vi "datacomb.vi"(0 "object in":refnum<class "212format_work.lvclass">, 1 "枚举":T1(ring), 5 "error in (no error)":errorcluster) -> (14 "object out":refnum<class "212format_work.lvclass">, 15 "字符串":string, 19 "error out":errorcluster)   [LabVIEW 2016, in "212format_work.lvclass"]
uses:
  212format_work.lvclass
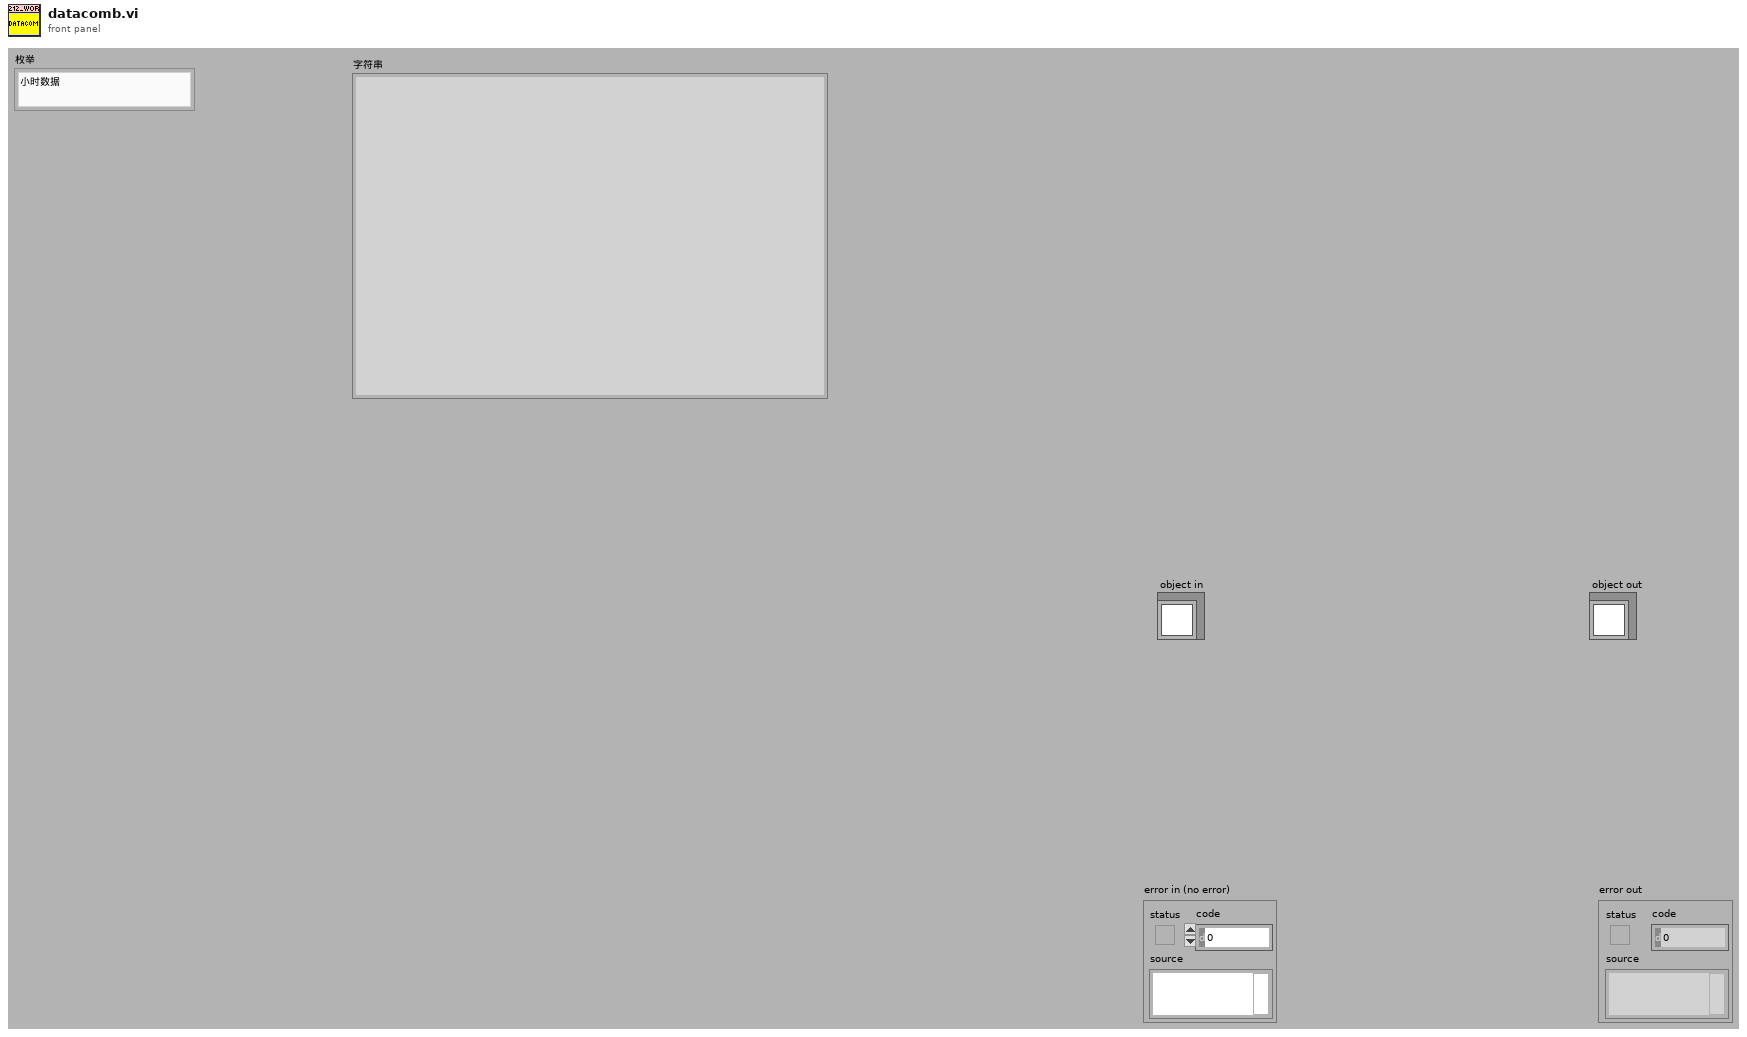
[diagram p1: front panel]
types:
  T1 = enum16{"小时数据", "实时数据", "平行样测试", "集成干预测试", "加标回收测试", "核查数据", "空白零点跨度数据", "提取小时数据", "提取实时数据", "操作日志", "仪器参数", "3090仪器参数", "提取仪器参数", "报警信息"}
  T2 = typedef "212format_work.lvclass/data控件.ctl" = cluster{"选择发送的参数":string, "插值后的数组元素":cluster{"PH":string[][], "CODCr":string[][], "氨氮":string[][], "CODMn":string[][], "总氮":string[][], "总磷":string[][], "电导率":string[][], "水温":string[][], "DO":string[][], "浊度":string[][], "叶绿素":string[][], "藻密度":string[][], "铜":string[][], "盐度":string[][], "水位":string[][], "流速":string[][], "瞬时流量":string[][], "累积流量":string[][], "亚硝酸盐":string[][], "硫化物":string[][], "ORP":string[][], "铅":string[][], "镉":string[][], "锌":string[][], "镍":string[][], "锰":string[][], "汞":string[][], "气温":string[][], "气压":string[][], "风速":string[][], "风向":string[][], "盐度 2":string[][], "磷酸盐":string[][], "硝氮":string[][], "氟化物":string[][], "挥发酚":string[][], "氯化物":string[][]}, "register values":u16[], "columns输出":string[], "环境参数":string[][], "仪器编码":string, "实时数据发送间隔":u32, "实时数据参数":string, "参数系数簇":cluster{"CODMn":dbl, "CODCr":dbl, "DO":dbl, "铜":dbl, "PH":dbl, "氨氮":dbl, "比电导率":dbl, "水温":dbl, "COD":dbl, "浊度":dbl, "总氮":dbl, "总磷":dbl, "叶绿素a":dbl, "藻密度":dbl, "水位":dbl, "流速":dbl, "瞬时流量":dbl, "累积流量":dbl, "亚硝酸盐":dbl, "硫化物":dbl, "ORP":dbl, "铅":dbl, "镉":dbl, "锌":dbl, "镍":dbl, "锰":dbl, "汞":dbl, "气温":dbl, "气压":dbl, "风速":dbl, "风向":dbl, "盐度":dbl, "磷酸盐":dbl, "硝氮":dbl, "氟化物":dbl, "挥发酚":dbl, "氯化物":dbl}, "因子编码簇":cluster{"CODMn":string, "CODCr":string, "DO":string, "铜":string, "PH":string, "氨氮":string, "比电导率":string, "水温":string, "COD":string, "浊度":string, "总氮":string, "总磷":string, "叶绿素a":string, "藻密度":string, "水位":string, "流速":string, "瞬时流量":string, "累积流量":string, "亚硝酸盐":string, "硫化物":string, "ORP":string, "铅":string, "镉":string, "锌":string, "镍":string, "锰":string, "汞":string, "气温":string, "气压":string, "风速":string, "风向":string, "盐度":string, "磷酸盐":string, "硝氮":string, "氟化物":string, "挥发酚":string, "氯化物":string}, "小时数据发送次数":i32, "读取试剂余量的值":u16[], "参数编码":string, "数据数组大小":i32, "总包数":i32, "当前包号":i32, "columns":string[], "剖面多参数":string[][], "分包标准":i32}
  T3 = cluster{"PH":string[][], "CODCr":string[][], "氨氮":string[][], "CODMn":string[][], "总氮":string[][], "总磷":string[][], "电导率":string[][], "水温":string[][], "DO":string[][], "浊度":string[][], "叶绿素":string[][], "藻密度":string[][], "铜":string[][], "盐度":string[][], "水位":string[][], "流速":string[][], "瞬时流量":string[][], "累积流量":string[][], "亚硝酸盐":string[][], "硫化物":string[][], "ORP":string[][], "铅":string[][], "镉":string[][], "锌":string[][], "镍":string[][], "锰":string[][], "汞":string[][], "气温":string[][], "气压":string[][], "风速":string[][], "风向":string[][], "盐度 2":string[][], "磷酸盐":string[][], "硝氮":string[][], "氟化物":string[][], "挥发酚":string[][], "氯化物":string[][]}
  T4 = cluster{"CODMn":dbl, "CODCr":dbl, "DO":dbl, "铜":dbl, "PH":dbl, "氨氮":dbl, "比电导率":dbl, "水温":dbl, "COD":dbl, "浊度":dbl, "总氮":dbl, "总磷":dbl, "叶绿素a":dbl, "藻密度":dbl, "水位":dbl, "流速":dbl, "瞬时流量":dbl, "累积流量":dbl, "亚硝酸盐":dbl, "硫化物":dbl, "ORP":dbl, "铅":dbl, "镉":dbl, "锌":dbl, "镍":dbl, "锰":dbl, "汞":dbl, "气温":dbl, "气压":dbl, "风速":dbl, "风向":dbl, "盐度":dbl, "磷酸盐":dbl, "硝氮":dbl, "氟化物":dbl, "挥发酚":dbl, "氯化物":dbl}
  T5 = cluster{"CODMn":string, "CODCr":string, "DO":string, "铜":string, "PH":string, "氨氮":string, "比电导率":string, "水温":string, "COD":string, "浊度":string, "总氮":string, "总磷":string, "叶绿素a":string, "藻密度":string, "水位":string, "流速":string, "瞬时流量":string, "累积流量":string, "亚硝酸盐":string, "硫化物":string, "ORP":string, "铅":string, "镉":string, "锌":string, "镍":string, "锰":string, "汞":string, "气温":string, "气压":string, "风速":string, "风向":string, "盐度":string, "磷酸盐":string, "硝氮":string, "氟化物":string, "挥发酚":string, "氯化物":string}
  T6 = typedef "212format_work.lvclass/interdata控件.ctl" = cluster{"数据发送协议":enum16{"2005-212协议", "2017-212协议"}, "枚举":enum16{"返回请求应答", "上传数据", "返回执行结果"}, "系统编码ST":string, "主动上报数据中":bool, "数据组合发送":bool, "地表水/污染源":bool, "应用环境":enum16{"STD", "GB212"}}
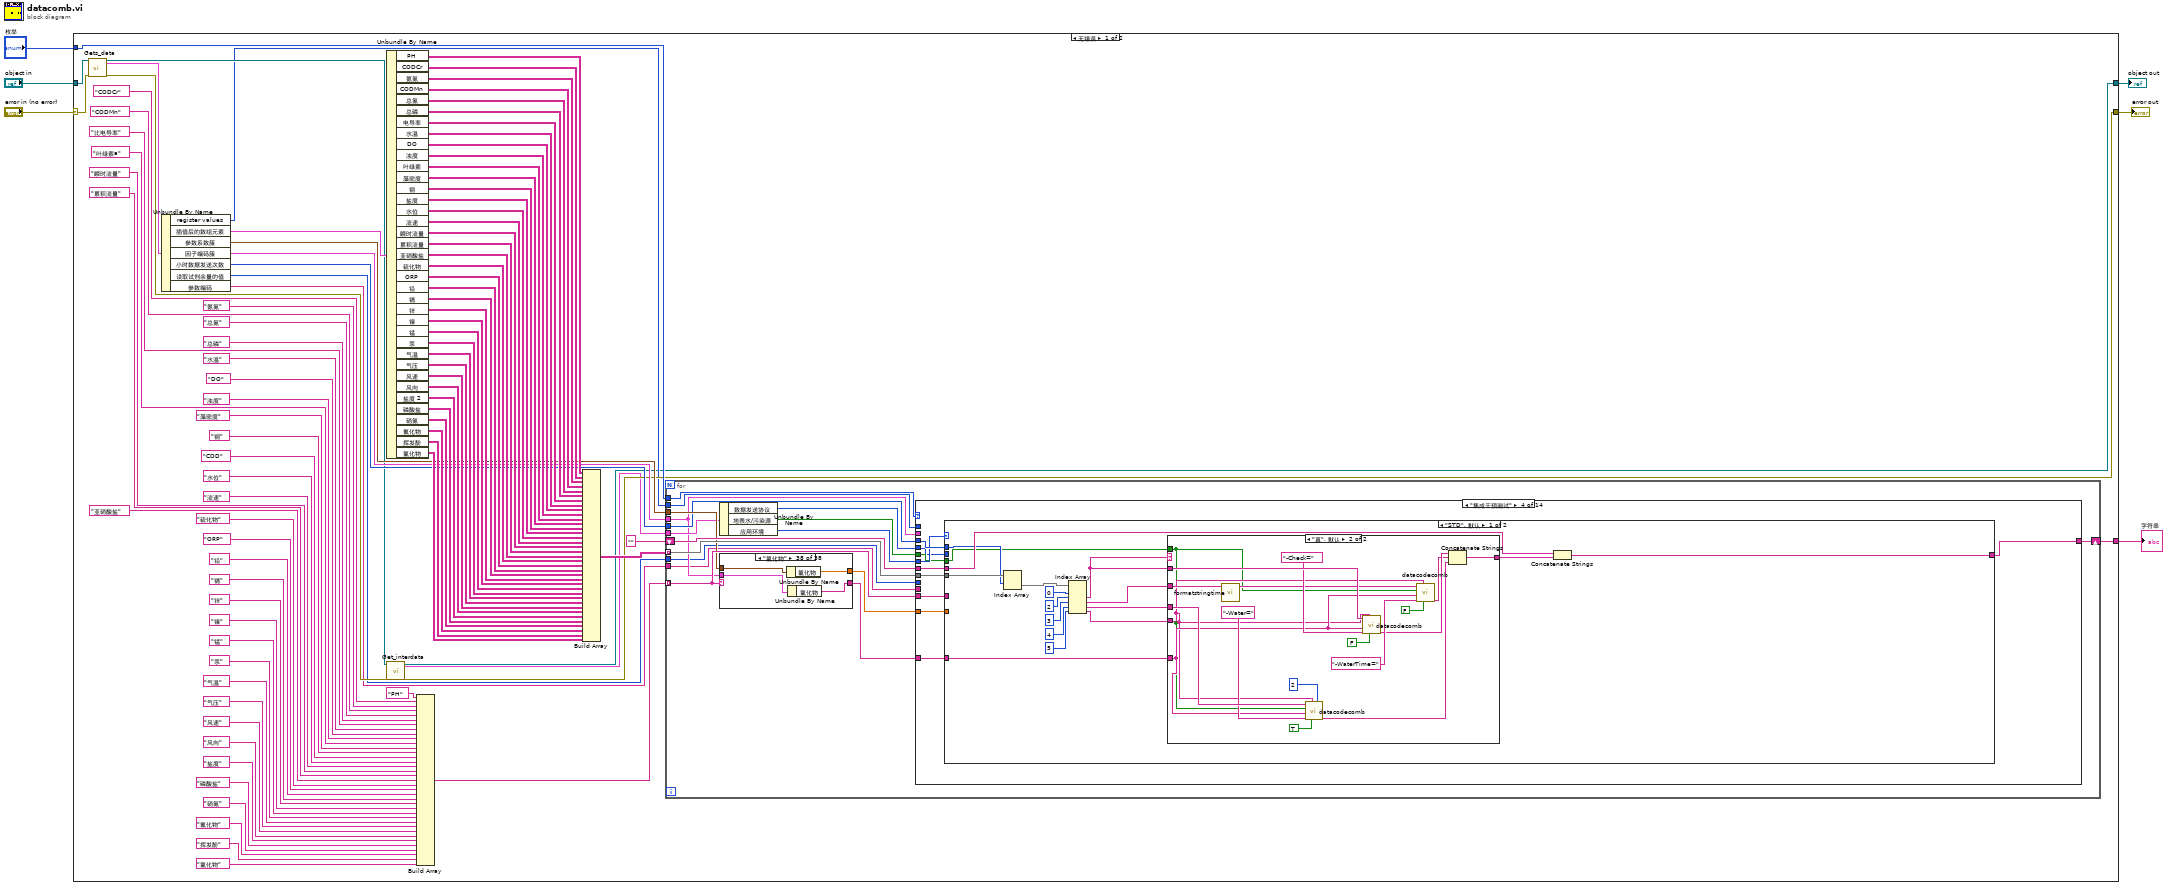
[diagram p0: block diagram]
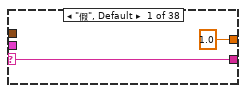
[diagram p2: hidden frame]
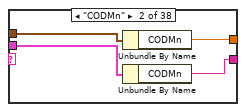
[diagram p3: hidden frame]
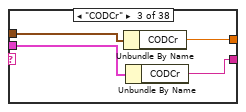
[diagram p4: hidden frame]
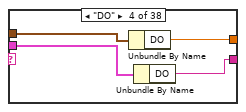
[diagram p5: hidden frame]
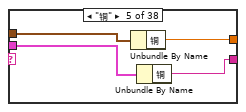
[diagram p6: hidden frame]
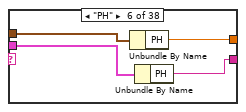
[diagram p7: hidden frame]
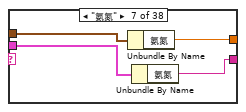
[diagram p8: hidden frame]
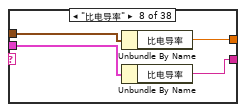
[diagram p9: hidden frame]
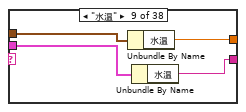
[diagram p10: hidden frame]
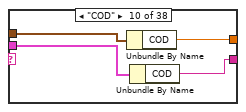
[diagram p11: hidden frame]
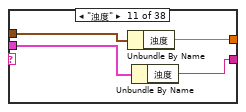
[diagram p12: hidden frame]
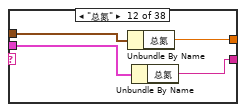
[diagram p13: hidden frame]
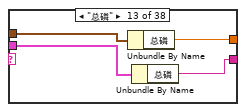
[diagram p14: hidden frame]
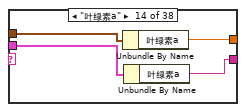
[diagram p15: hidden frame]
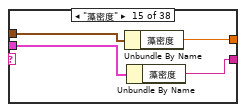
[diagram p16: hidden frame]
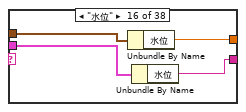
[diagram p17: hidden frame]
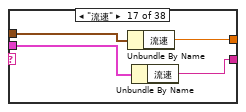
[diagram p18: hidden frame]
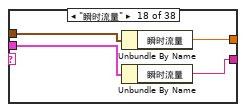
[diagram p19: hidden frame]
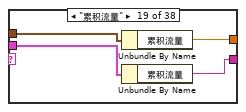
[diagram p20: hidden frame]
diagram:
  n1 = case shown="无错误" "error in (no error)" {
    selector: "error in (no error)" -> [w19 w841]
    tunnel: [w13 w841] -> w5
    tunnel: [w7 w840] -> w3
    tunnel: "object in" -> [w20 w840]
    tunnel: "枚举" -> [w23 _]
    tunnel: [w11 _] -> w1
    frame No Error {
      n2 = call-dynamic "Gets_data.vi"("object in"=w20, "error in (no error)"=w19) -> ("object out"=w15:refnum<class "212format_work.lvclass">, "data"=w22:T2, "error out"=w14:errorcluster)  [unwired: 15 in]
      n3 = Unbundle By Name(w22) -> ("register values"=w10:u16[], "插值后的数组元素"=w21:T3, "参数系数簇"=w18:T4, "因子编码簇"=w17:T5, "小时数据发送次数"=w16:i32, "读取试剂余量的值"=w9:u16[], "参数编码"=w8:string)
      n4 = Unbundle By Name(w21) -> ("PH"=w100:string[][], "CODCr"=w99:string[][], "氨氮"=w98:string[][], "CODMn"=w97:string[][], "总氮"=w96:string[][], "总磷"=w95:string[][], "电导率"=w94:string[][], "水温"=w93:string[][], "DO"=w92:string[][], "浊度"=w91:string[][], "叶绿素"=w90:string[][], "藻密度"=w89:string[][], "铜"=w88:string[][], "盐度"=w87:string[][], "水位"=w86:string[][], "流速"=w85:string[][], "瞬时流量"=w84:string[][], "累积流量"=w83:string[][], "亚硝酸盐"=w82:string[][], "硫化物"=w81:string[][], "ORP"=w80:string[][], "铅"=w79:string[][], "镉"=w78:string[][], "锌"=w77:string[][], "镍"=w76:string[][], "锰"=w75:string[][], "汞"=w74:string[][], "气温"=w40:string[][], "气压"=w41:string[][], "风速"=w42:string[][], "风向"=w43:string[][], "盐度 2"=w35:string[][], "磷酸盐"=w34:string[][], "硝氮"=w33:string[][], "氟化物"=w29:string[][], "挥发酚"=w27:string[][], "氯化物"=w26:string[][])
      n5 = call-dynamic "Get_interdata.vi"("object in"=w15, "error in (no error)"=w14) -> ("object out"=w7:refnum<class "212format_work.lvclass">, "interdata"=w12:T6, "error out"=w13:errorcluster)  [unwired: 15 in]
      n6 = Build Array("PH" ("污染物编码"), "CODCr" ("污染物编码"), "氨氮" ("污染物编码"), "CODMn" ("污染物编码"), "总氮" ("污染物编码"), "总磷" ("污染物编码"), "比电导率" ("污染物编码"), "水温" ("污染物编码"), "DO" ("污染物编码"), "浊度" ("污染物编码"), "叶绿素a" ("污染物编码"), "藻密度" ("污染物编码"), "铜" ("污染物编码"), "COD" ("污染物编码"), "水位" ("污染物编码"), "流速" ("污染物编码"), "瞬时流量" ("污染物编码"), "累积流量" ("污染物编码"), "亚硝酸盐" ("污染物编码"), "硫化物" ("污染物编码"), "ORP" ("污染物编码"), "铅" ("污染物编码"), "镉" ("污染物编码"), "锌" ("污染物编码"), "镍" ("污染物编码"), "锰" ("污染物编码"), "汞" ("污染物编码"), "气温" ("污染物编码"), "气压" ("污染物编码"), "风速" ("污染物编码"), "风向" ("污染物编码"), "盐度" ("污染物编码"), "磷酸盐" ("污染物编码"), "硝氮" ("污染物编码"), "氟化物" ("污染物编码"), "挥发酚" ("污染物编码"), "氯化物" ("污染物编码")) -> (w45:string[])
      n7 = Build Array(w100, w99, w98, w97, w96, w95, w94, w93, w92, w91, w90, w89, w88, w87, w86, w85, w84, w83, w82, w81, w80, w79, w78, w77, w76, w75, w74, w40, w41, w42, w43, w35, w34, w33, w29, w27, w26) -> (w73:string[][][])
      n8 = for {
        tunnel: w73 -> [w117] mode=indexing
        tunnel: w45 -> [w112] mode=indexing
        shift-right: [w116] -> w11
        shift-left: "" -> [w115]
        tunnel: w23 -> [w114]
        tunnel: w18 -> [w110]
        tunnel: w17 -> [w104]
        tunnel: w16 -> [w109]
        tunnel: w12 -> [w108]
        tunnel: w10 -> [w103]
        tunnel: w9 -> [w102]
        tunnel: w8 -> [w101]
        n9 = Unbundle By Name(w108) -> ("数据发送协议"=w106:enum16{"2005-212协议", "2017-212协议"}, "地表水/污染源"=w107:bool, "应用环境"=w105:enum16{"STD", "GB212"})
        n10 = case shown="\"氯化物\"" w112 {
          selector: w112 -> [w119 _ _ _ _ _ _ _ _ _ _ _ _ _ _ _ _ _ _ _ _ _ _ _ _ _ _ _ _ _ _ _ _ _ _ _ _ _]
          tunnel: [w119 w123 w127 w131 w135 w139 w143 w147 w151 w155 w159 w163 w167 w171 w175 w179 w183 w187 w191 w195 w199 w203 w207 w211 w215 w219 w223 w227 w231 w235 w239 w243 w247 w251 w255 w259 w263 w267] -> w113
          tunnel: [1.0 ("风向") w122 w126 w130 w134 w138 w142 w146 w150 w154 w158 w162 w166 w170 w174 w178 w182 w186 w190 w194 w198 w202 w206 w210 w214 w218 w222 w226 w230 w234 w238 w242 w246 w250 w254 w258 w262 w266] -> w111
          tunnel: w110 -> [_ w121 w125 w129 w133 w137 w141 w145 w149 w153 w157 w161 w165 w169 w173 w177 w181 w185 w189 w193 w197 w201 w205 w209 w213 w217 w221 w225 w229 w233 w237 w241 w245 w249 w253 w257 w261 w265]
          tunnel: w104 -> [_ w120 w124 w128 w132 w136 w140 w144 w148 w152 w156 w160 w164 w168 w172 w176 w180 w184 w188 w192 w196 w200 w204 w208 w212 w216 w220 w224 w228 w232 w236 w240 w244 w248 w252 w256 w260 w264]
          frame "假", Default {
          }
          frame "CODMn" {
            n11 = Unbundle By Name(w121) -> ("CODMn"=w122:dbl)
            n12 = Unbundle By Name(w120) -> ("CODMn"=w123:string)
          }
          frame "CODCr" {
            n13 = Unbundle By Name(w125) -> ("CODCr"=w126:dbl)
            n14 = Unbundle By Name(w124) -> ("CODCr"=w127:string)
          }
          frame "DO" {
            n15 = Unbundle By Name(w129) -> ("DO"=w130:dbl)
            n16 = Unbundle By Name(w128) -> ("DO"=w131:string)
          }
          frame "铜" {
            n17 = Unbundle By Name(w133) -> ("铜"=w134:dbl)
            n18 = Unbundle By Name(w132) -> ("铜"=w135:string)
          }
          frame "PH" {
            n19 = Unbundle By Name(w137) -> ("PH"=w138:dbl)
            n20 = Unbundle By Name(w136) -> ("PH"=w139:string)
          }
          frame "氨氮" {
            n21 = Unbundle By Name(w141) -> ("氨氮"=w142:dbl)
            n22 = Unbundle By Name(w140) -> ("氨氮"=w143:string)
          }
          frame "比电导率" {
            n23 = Unbundle By Name(w145) -> ("比电导率"=w146:dbl)
            n24 = Unbundle By Name(w144) -> ("比电导率"=w147:string)
          }
          frame "水温" {
            n25 = Unbundle By Name(w149) -> ("水温"=w150:dbl)
            n26 = Unbundle By Name(w148) -> ("水温"=w151:string)
          }
          frame "COD" {
            n27 = Unbundle By Name(w153) -> ("COD"=w154:dbl)
            n28 = Unbundle By Name(w152) -> ("COD"=w155:string)
          }
          frame "浊度" {
            n29 = Unbundle By Name(w157) -> ("浊度"=w158:dbl)
            n30 = Unbundle By Name(w156) -> ("浊度"=w159:string)
          }
          frame "总氮" {
            n31 = Unbundle By Name(w161) -> ("总氮"=w162:dbl)
            n32 = Unbundle By Name(w160) -> ("总氮"=w163:string)
          }
          frame "总磷" {
            n33 = Unbundle By Name(w165) -> ("总磷"=w166:dbl)
            n34 = Unbundle By Name(w164) -> ("总磷"=w167:string)
          }
          frame "叶绿素a" {
            n35 = Unbundle By Name(w169) -> ("叶绿素a"=w170:dbl)
            n36 = Unbundle By Name(w168) -> ("叶绿素a"=w171:string)
          }
          frame "藻密度" {
            n37 = Unbundle By Name(w173) -> ("藻密度"=w174:dbl)
            n38 = Unbundle By Name(w172) -> ("藻密度"=w175:string)
          }
          frame "水位" {
            n39 = Unbundle By Name(w177) -> ("水位"=w178:dbl)
            n40 = Unbundle By Name(w176) -> ("水位"=w179:string)
          }
          frame "流速" {
            n41 = Unbundle By Name(w181) -> ("流速"=w182:dbl)
            n42 = Unbundle By Name(w180) -> ("流速"=w183:string)
          }
          frame "瞬时流量" {
            n43 = Unbundle By Name(w185) -> ("瞬时流量"=w186:dbl)
            n44 = Unbundle By Name(w184) -> ("瞬时流量"=w187:string)
          }
          frame "累积流量" {
            n45 = Unbundle By Name(w189) -> ("累积流量"=w190:dbl)
            n46 = Unbundle By Name(w188) -> ("累积流量"=w191:string)
          }
          frame "亚硝酸盐" {
            n47 = Unbundle By Name(w193) -> ("亚硝酸盐"=w194:dbl)
            n48 = Unbundle By Name(w192) -> ("亚硝酸盐"=w195:string)
          }
          frame "硫化物" {
            n49 = Unbundle By Name(w197) -> ("硫化物"=w198:dbl)
            n50 = Unbundle By Name(w196) -> ("硫化物"=w199:string)
          }
          frame "ORP" {
            n51 = Unbundle By Name(w201) -> ("ORP"=w202:dbl)
            n52 = Unbundle By Name(w200) -> ("ORP"=w203:string)
          }
          frame "铅" {
            n53 = Unbundle By Name(w205) -> ("铅"=w206:dbl)
            n54 = Unbundle By Name(w204) -> ("铅"=w207:string)
          }
          frame "镉" {
            n55 = Unbundle By Name(w209) -> ("镉"=w210:dbl)
            n56 = Unbundle By Name(w208) -> ("镉"=w211:string)
          }
          frame "锌" {
            n57 = Unbundle By Name(w213) -> ("锌"=w214:dbl)
            n58 = Unbundle By Name(w212) -> ("锌"=w215:string)
          }
          frame "镍" {
            n59 = Unbundle By Name(w217) -> ("镍"=w218:dbl)
            n60 = Unbundle By Name(w216) -> ("镍"=w219:string)
          }
          frame "锰" {
            n61 = Unbundle By Name(w221) -> ("锰"=w222:dbl)
            n62 = Unbundle By Name(w220) -> ("锰"=w223:string)
          }
          frame "汞" {
            n63 = Unbundle By Name(w225) -> ("汞"=w226:dbl)
            n64 = Unbundle By Name(w224) -> ("汞"=w227:string)
          }
          frame "气温" {
            n65 = Unbundle By Name(w229) -> ("气温"=w230:dbl)
            n66 = Unbundle By Name(w228) -> ("气温"=w231:string)
          }
          frame "气压" {
            n67 = Unbundle By Name(w233) -> ("气压"=w234:dbl)
            n68 = Unbundle By Name(w232) -> ("气压"=w235:string)
          }
          frame "风速" {
            n69 = Unbundle By Name(w237) -> ("风速"=w238:dbl)
            n70 = Unbundle By Name(w236) -> ("风速"=w239:string)
          }
          frame "风向" {
            n71 = Unbundle By Name(w241) -> ("风向"=w242:dbl)
            n72 = Unbundle By Name(w240) -> ("风向"=w243:string)
          }
          frame "盐度" {
            n73 = Unbundle By Name(w245) -> ("盐度"=w246:dbl)
            n74 = Unbundle By Name(w244) -> ("盐度"=w247:string)
          }
          frame "磷酸盐" {
            n75 = Unbundle By Name(w249) -> ("磷酸盐"=w250:dbl)
            n76 = Unbundle By Name(w248) -> ("磷酸盐"=w251:string)
          }
          frame "硝氮" {
            n77 = Unbundle By Name(w253) -> ("硝氮"=w254:dbl)
            n78 = Unbundle By Name(w252) -> ("硝氮"=w255:string)
          }
          frame "氟化物" {
            n79 = Unbundle By Name(w257) -> ("氟化物"=w258:dbl)
            n80 = Unbundle By Name(w256) -> ("氟化物"=w259:string)
          }
          frame "挥发酚" {
            n81 = Unbundle By Name(w261) -> ("挥发酚"=w262:dbl)
            n82 = Unbundle By Name(w260) -> ("挥发酚"=w263:string)
          }
          frame "氯化物" {
            n83 = Unbundle By Name(w265) -> ("氯化物"=w266:dbl)
            n84 = Unbundle By Name(w264) -> ("氯化物"=w267:string)
          }
        }
        n85 = case shown="\"集成干预测试\"" w114 {
          tunnel: w117 -> [w281 w327 w358 w398 w481 w524 w574 w596 w619 w655 w673 w681 w695 w781]
          tunnel: w113 -> [w278 w321 w356 w399 w480 w522 w561 w591 w618 w644 w671 w679 w685 w783]
          tunnel: [w280 w324 w369 w396 w519 w533 w572 w588 w617 w650 w668 w678 w693 w769] -> w116
          tunnel: w115 -> [w279 w325 w370 w397 w518 w534 w573 w589 w620 w651 w669 w680 w694 w764]
          tunnel: w112 -> [w275 w320 _ w394 _ _ _ _ _ _ _ _ _ w779]
          tunnel: w111 -> [w272 w316 _ w395 _ _ _ w584 w613 _ _ _ _ _]
          tunnel: w109 -> [w270 w315 w357 w393 w482 w523 w550 w583 w610 w641 w666 w677 w692 w760]
          tunnel: w107 -> [w269 w313 w354 w391 _ w520 w554 w582 w612 _ _ _ _ _]
          tunnel: w106 -> [w268 w314 _ w390 _ _ _ w581 w611 _ _ _ _ _]
          tunnel: w105 -> [_ _ _ w392 _ _ _ _ _ _ w665 w676 _ _]
          tunnel: w104 -> [_ _ _ _ _ _ _ _ _ w640 _ _ _ w759]
          tunnel: w103 -> [_ _ _ _ _ _ _ _ _ _ _ _ _ w758]
          tunnel: w102 -> [_ _ _ _ _ _ _ _ _ _ _ _ _ w757]
          tunnel: w101 -> [_ _ _ _ _ _ _ _ _ _ _ _ w687 _]
          frame "小时数据", Default {
            n86 = Index Array(array=w281, index (row)=w270) -> (element=w284:string[])  [unwired: 1 in]
            n87 = case shown="\"风速\", \"风向\", \"累积流量\", \"流速\", \"气温\", \"气压\", \"水位\", \"瞬时流量\"" w275 {
              tunnel: w284 -> [w294 w297]
              tunnel: [w291 w296] -> w273
              tunnel: ["N" ("字符串") w295] -> w282
              frame "风速", "风向", "累积流量", "流速", "气温", "气压", "水位", "瞬时流量" {
                n88 = Index Array(array=w294, index=1 ("索引")) -> (element=w291:string)
              }
              frame "", Default {
                n89 = Index Array(array=w297, index #1=2 ("索引"), index #2=3 ("索引"), index #3=5 ("索引")) -> (element #1=w300:string, element #2=w299:string, element #3=w295:string)
                n90 = case shown="\"N\", 默认" w300 {
                  tunnel: [w303 ""] -> w296
                  tunnel: w299 -> [w303 _]
                  frame "N", Default {
                  }
                  frame "M" {
                  }
                }
              }
            }
            n91 = Empty String/Path?(string/path=w273) -> (empty?=w274:bool)
            n92 = case shown="假" w274 {
              tunnel: w273 -> [w288 w290]
              tunnel: w272 -> [w287 _]
              tunnel: [w285 w290] -> w271
              frame False {
                n93 = Fract/Exp String To Number(string=w288) -> (number=w289:dbl)  [unwired: 3 in, 1 out]
                n94 = Multiply(x=w289, y=w287) -> (x*y=w286:dbl)
                n95 = Number To Fractional String(number=w286) -> (F-format string=w285:string)  [unwired: 3 in]
              }
              frame True {
                # "空"
              }
            }
            n96 = call "datacodecomb.vi"("数据标识"=w282, "数据类型"="-Avg=", "污染物编码"=w278, "地表水/污染源"=w269, "污染物浓度"=w271) -> ("编码输出"=w277:string)  [unwired: 6 in]
            n97 = case shown="\"2005-212协议\", 默认" w268 {
              tunnel: w275 -> [w307 _]
              tunnel: w277 -> [w305 w310]
              tunnel: [w306 w310] -> w276
              frame "2005-212协议", Default {
                n98 = case shown="\"风速\", \"风向\", \"累积流量\", \"流速\", \"气温\", \"气压\", \"水位\"" w307 {
                  tunnel: [w308 ""] -> w306
                  tunnel: w305 -> [w308 _]
                  frame "假", Default {
                  }
                  frame "风速", "风向", "累积流量", "流速", "气温", "气压", "水位" {
                  }
                }
              }
              frame "2017-212协议" {
              }
            }
            n99 = Concatenate Strings(w279, w276) -> (w280:string)
          }
          frame "实时数据" {
            n100 = Index Array(array=w327, index (row)=w315) -> (element=w312:string[])  [unwired: 1 in]
            n101 = case shown="\"累积流量\", \"流速\", \"水位\", \"瞬时流量\"" w320 {
              tunnel: w312 -> [w336 w340 w346]
              tunnel: [w335 w339 w345] -> w318
              tunnel: ["N" ("字符串") "N" ("字符串") w343] -> w326
              frame "累积流量", "流速", "水位", "瞬时流量" {
                n102 = Index Array(array=w336, index=1 ("索引")) -> (element=w335:string)
              }
              frame "风速", "风向", "气温", "气压" {
                n103 = Index Array(array=w340, index=1 ("索引")) -> (element=w339:string)
              }
              frame "", Default {
                n104 = Index Array(array=w346, index #1=3 ("索引"), index #2=5 ("索引")) -> (element #1=w345:string, element #2=w343:string)
              }
            }
            n105 = Empty String/Path?(string/path=w318) -> (empty?=w319:bool)
            n106 = case shown="假" w319 {
              tunnel: w318 -> [w332 w334]
              tunnel: w316 -> [w331 _]
              tunnel: [w329 w334] -> w317
              frame False {
                n107 = Fract/Exp String To Number(string=w332) -> (number=w333:dbl)  [unwired: 3 in, 1 out]
                n108 = Multiply(x=w333, y=w331) -> (x*y=w330:dbl)
                n109 = Number To Fractional String(number=w330) -> (F-format string=w329:string)  [unwired: 3 in]
              }
              frame True {
                # "空"
              }
            }
            n110 = Index Array(array=w312) -> (element=w311:string)  [unwired: 1 in]
            n111 = Empty String/Path?(string/path=w311) -> ()  [unwired: 1 out]
            n112 = call "datacodecomb.vi"("数据标识"=w326, "数据类型"="-Rtd=", "污染物编码"=w321, "地表水/污染源"=w313, "污染物浓度"=w317) -> ("编码输出"=w323:string)  [unwired: 6 in]
            n113 = case shown="\"2017-212协议\"" w314 {
              tunnel: w320 -> [w350 _]
              tunnel: w323 -> [w348 w353]
              tunnel: [w349 w353] -> w322
              frame "2005-212协议", Default {
                n114 = case shown="\"假\", 默认" w350 {
                  tunnel: [w351 ""] -> w349
                  tunnel: w348 -> [w351 _]
                  frame "假", Default {
                  }
                  frame "风速", "风向", "累积流量", "流速", "气温", "气压", "水位" {
                  }
                }
              }
              frame "2017-212协议" {
              }
            }
            n115 = Concatenate Strings(w325, w322) -> (w324:string)
          }
          frame "平行样测试" {
            n116 = Index Array(array=w358, index (row)=w357) -> (element=w365:string[])  [unwired: 1 in]
            n117 = Index Array(array=w365, index #1=0 ("索引"), index #2=2 ("索引"), index #3=3 ("索引"), index #4=4 ("索引"), index #5=5 ("索引")) -> (element #2=w362:string, element #3=w364:string, element #4=w363:string, element #5=w359:string)  [unwired: 1 out]
            n118 = case shown="\"真\", 默认" w362 {
              selector: w362 -> [w371 _]
              tunnel: w362 -> [_ w389]
              tunnel: w363 -> [_ w383]
              tunnel: w364 -> [_ w381]
              tunnel: [w371 w376] -> w355
              tunnel: w356 -> [_ w375]
              tunnel: w359 -> [_ w373]
              tunnel: w354 -> [_ w372]
              frame "" {
              }
              frame "真", Default {
                n119 = call "formatstringtime.vi"("字符串"=w381) -> ("result string"=w380:string)  [unwired: 10 in]
                n120 = call "datacodecomb.vi"("数据精度"=2, "字段结束"=TRUE, "数据标识"=w373, "数据类型"="-Water=", "污染物编码"=w375, "地表水/污染源"=w372, "污染物浓度"=w383) -> ("编码输出"=w377:string)  [unwired: 4 in]
                n121 = call "datacodecomb.vi"("字段结束"=FALSE, "数据标识"=w373, "数据类型"="-Check=", "污染物编码"=w375, "地表水/污染源"=w372, "污染物浓度"=w389) -> ("编码输出"=w379:string)  [unwired: 5 in]
                n122 = call "datacodecomb.vi"("字段结束"=FALSE, "数据标识"=w373, "数据类型"="-WaterTime=", "污染物编码"=w375, "地表水/污染源"=w372, "污染物浓度"=w380) -> ("编码输出"=w378:string)  [unwired: 5 in]
                n123 = Concatenate Strings(w379, w378, w377) -> (w376:string)
              }
            }
            n124 = Concatenate Strings(w370, w355) -> (w369:string)
          }
          frame "集成干预测试" {
            n125 = case shown="\"STD\", 默认" w392 {
              tunnel: w399 -> [w402 w442]
              tunnel: w398 -> [w404 w443]
              tunnel: w397 -> [w416 w444]
              tunnel: [w415 w439] -> w396
              tunnel: w395 -> [_ w441]
              tunnel: w394 -> [_ w440]
              tunnel: w393 -> [w403 w438]
              tunnel: w391 -> [w401 w437]
              tunnel: w390 -> [_ w436]
              frame "STD", Default {
                n126 = Index Array(array=w404, index (row)=w403) -> (element=w411:string[])  [unwired: 1 in]
                n127 = Index Array(array=w411, index #1=0 ("索引"), index #2=2 ("索引"), index #3=3 ("索引"), index #4=4 ("索引"), index #5=5 ("索引")) -> (element #2=w408:string, element #3=w410:string, element #4=w409:string, element #5=w405:string)  [unwired: 1 out]
                n128 = case shown="\"真\", 默认" w408 {
                  selector: w408 -> [w417 _]
                  tunnel: w408 -> [_ w435]
                  tunnel: w409 -> [_ w429]
                  tunnel: w410 -> [_ w427]
                  tunnel: [w417 w422] -> w400
                  tunnel: w402 -> [_ w421]
                  tunnel: w405 -> [_ w419]
                  tunnel: w401 -> [_ w418]
                  frame "" {
                  }
                  frame "真", Default {
                    n129 = call "formatstringtime.vi"("字符串"=w427) -> ("result string"=w426:string)  [unwired: 10 in]
                    n130 = call "datacodecomb.vi"("数据精度"=2, "字段结束"=TRUE, "数据标识"=w419, "数据类型"="-Water=", "污染物编码"=w421, "地表水/污染源"=w418, "污染物浓度"=w429) -> ("编码输出"=w423:string)  [unwired: 4 in]
                    n131 = call "datacodecomb.vi"("字段结束"=FALSE, "数据标识"=w419, "数据类型"="-Check=", "污染物编码"=w421, "地表水/污染源"=w418, "污染物浓度"=w435) -> ("编码输出"=w425:string)  [unwired: 5 in]
                    n132 = call "datacodecomb.vi"("字段结束"=FALSE, "数据标识"=w419, "数据类型"="-WaterTime=", "污染物编码"=w421, "地表水/污染源"=w418, "污染物浓度"=w426) -> ("编码输出"=w424:string)  [unwired: 5 in]
                    n133 = Concatenate Strings(w425, w424, w423) -> (w422:string)
                  }
                }
                n134 = Concatenate Strings(w416, w400) -> (w415:string)
              }
              frame "GB212" {
                n135 = Index Array(array=w443, index (row)=w438) -> (element=w452:string[])  [unwired: 1 in]
                n136 = case shown="\"\", 默认" w440 {
                  tunnel: w452 -> [w462 w465]
                  tunnel: [w459 w464] -> w446
                  tunnel: ["N" ("字符串") w463] -> w450
                  frame "风速", "风向", "累积流量", "流速", "气温", "气压", "水位", "瞬时流量" {
                    n137 = Index Array(array=w462, index=1 ("索引")) -> (element=w459:string)
                  }
                  frame "", Default {
                    n138 = Index Array(array=w465, index #1=2 ("索引"), index #2=3 ("索引"), index #3=5 ("索引")) -> (element #1=w468:string, element #2=w467:string, element #3=w463:string)
                    n139 = case shown="\"N\", 默认" w468 {
                      tunnel: [w471 ""] -> w464
                      tunnel: w467 -> [w471 _]
                      frame "N", Default {
                      }
                      frame "M" {
                      }
                    }
                  }
                }
                n140 = Empty String/Path?(string/path=w446) -> (empty?=w447:bool)
                n141 = case shown="假" w447 {
                  tunnel: w446 -> [w456 w458]
                  tunnel: w441 -> [w455 _]
                  tunnel: [w453 w458] -> w445
                  frame False {
                    n142 = Fract/Exp String To Number(string=w456) -> (number=w457:dbl)  [unwired: 3 in, 1 out]
                    n143 = Multiply(x=w457, y=w455) -> (x*y=w454:dbl)
                    n144 = Number To Fractional String(number=w454) -> (F-format string=w453:string)  [unwired: 3 in]
                  }
                  frame True {
                    # "空"
                  }
                }
                n145 = call "datacodecomb.vi"("数据标识"=w450, "数据类型"="-Avg=", "污染物编码"=w442, "地表水/污染源"=w437, "污染物浓度"=w445) -> ("编码输出"=w449:string)  [unwired: 6 in]
                n146 = case shown="\"2017-212协议\"" w436 {
                  tunnel: w440 -> [w475 _]
                  tunnel: w449 -> [w473 w478]
                  tunnel: [w474 w478] -> w448
                  frame "2005-212协议", Default {
                    n147 = case shown="\"假\", 默认" w475 {
                      tunnel: [w476 ""] -> w474
                      tunnel: w473 -> [w476 _]
                      frame "假", Default {
                      }
                      frame "风速", "风向", "累积流量", "流速", "气温", "气压", "水位" {
                      }
                    }
                  }
                  frame "2017-212协议" {
                  }
                }
                n148 = Concatenate Strings(w444, w448) -> (w439:string)
              }
            }
          }
          frame "加标回收测试" {
            n149 = Index Array(array=w481, index (row)=w482) -> (element=w485:string[])  [unwired: 1 in]
            n150 = Index Array(array=w485, index #1=0 ("索引"), index #2=4 ("索引"), index #3=2 ("索引"), index #4=3 ("索引"), index #5=5 ("索引"), index #6=6 ("索引"), index #7=7 ("索引")) -> (element #2=w488:string, element #3=w516:string, element #4=w494:string, element #5=w496:string, element #6=w499:string, element #7=w500:string)  [unwired: 1 out]
            n151 = call "formatstringtime.vi"("字符串"=w516) -> ("result string"=w517:string)  [unwired: 10 in]
            n152 = call "datacodecomb.vi"("字段结束"=FALSE, "数据类型"="-Chroma=", "污染物编码"=w480, "污染物浓度"=w496) -> ("编码输出"=w506:string)  [unwired: 7 in]
            n153 = call "datacodecomb.vi"("字段结束"=FALSE, "数据类型"="-Volume=", "污染物编码"=w480, "污染物浓度"=w499) -> ("编码输出"=w507:string)  [unwired: 7 in]
            n154 = call "datacodecomb.vi"("字段结束"=TRUE, "数据类型"="-DVolume=", "污染物编码"=w480, "污染物浓度"=w500) -> ("编码输出"=w508:string)  [unwired: 7 in]
            n155 = call "datacodecomb.vi"("字段结束"=FALSE, "数据标识"="N" ("字符串"), "数据类型"="-Check=", "污染物编码"=w480, "污染物浓度"=w488) -> ("编码输出"=w503:string)  [unwired: 6 in]
            n156 = call "datacodecomb.vi"("数据精度"=2, "字段结束"=FALSE, "数据类型"="-Water=", "污染物编码"=w480, "污染物浓度"=w494) -> ("编码输出"=w505:string)  [unwired: 6 in]
            n157 = call "datacodecomb.vi"("字段结束"=FALSE, "数据类型"="-WaterTime=", "污染物编码"=w480, "污染物浓度"=w517) -> ("编码输出"=w504:string)  [unwired: 7 in]
            n158 = Concatenate Strings(w503, w504, w505, w506, w507, w508) -> (w479:string)
            n159 = Concatenate Strings(w518, w479) -> (w519:string)
          }
          frame "核查数据" {
            n160 = Index Array(array=w524, index (row)=w523) -> (element=w532:string[])  [unwired: 1 in]
            n161 = Index Array(array=w532, index #1=0 ("索引"), index #2=3 ("索引"), index #3=5 ("索引"), index #4=6 ("索引")) -> (element #2=w531:string, element #3=w525:string, element #4=w528:string)  [unwired: 1 out]
            n162 = case shown="\"真\", 默认" w531 {
              tunnel: w531 -> [w535 w549]
              tunnel: [w535 w546] -> w521
              tunnel: w528 -> [_ w543]
              tunnel: w522 -> [_ w539]
              tunnel: w525 -> [_ w538]
              tunnel: w520 -> [_ w536]
              frame "" {
              }
              frame "真", Default {
                n163 = call "datacodecomb.vi"("数据精度"=6, "字段结束"=FALSE, "数据标识"=w538, "数据类型"="-Check=", "污染物编码"=w539, "地表水/污染源"=w536, "污染物浓度"=w549) -> ("编码输出"=w547:string)  [unwired: 4 in]
                n164 = call "datacodecomb.vi"("数据精度"=2, "字段结束"=TRUE, "数据标识"=w538, "数据类型"="-StandardValue=", "污染物编码"=w539, "地表水/污染源"=w536, "污染物浓度"=w543) -> ("编码输出"=w544:string)  [unwired: 4 in]
                n165 = Concatenate Strings(w547, w544) -> (w546:string)
              }
            }
            n166 = Concatenate Strings(w534, w521) -> (w533:string)
          }
          frame "空白零点跨度数据" {
            w558 = 2 ("数据精度")
            w564 = FALSE ("字段结束")
            n167 = Index Array(array=w574, index (row)=w550) -> (element=w577:string[])  [unwired: 1 in]
            n168 = Index Array(array=w577, index #1=0 ("索引"), index #2=3 ("索引"), index #3=6 ("索引"), index #4=7 ("索引"), index #5=5 ("索引")) -> (element #2=w562:string, element #3=w552:string, element #4=w569:string, element #5=w563:string)  [unwired: 1 out]
            n169 = call "datacodecomb.vi"("数据精度"=w558, "字段结束"=w564, "数据标识"=w563, "数据类型"="-StandardValue=", "污染物编码"=w561, "地表水/污染源"=w554, "污染物浓度"=w552) -> ("编码输出"=w556:string)  [unwired: 4 in]
            n170 = Empty String/Path?(string/path=w569) -> (empty?=w570:bool)
            n171 = call "datacodecomb.vi"("数据精度"=6, "字段结束"=w564, "数据标识"=w563, "数据类型"="-Check=", "污染物编码"=w561, "地表水/污染源"=w554, "污染物浓度"=w562) -> ("编码输出"=w557:string)  [unwired: 4 in]
            n172 = case shown="假" w570 {
              tunnel: [w579 "0" ("span value")] -> w551
              tunnel: w569 -> [w579 _]
              frame False {
              }
              frame True {
              }
            }
            n173 = call "datacodecomb.vi"("数据精度"=w558, "字段结束"=TRUE, "数据标识"=w563, "数据类型"="-SpanValue=", "污染物编码"=w561, "地表水/污染源"=w554, "污染物浓度"=w551) -> ("编码输出"=w555:string)  [unwired: 4 in]
            n174 = Concatenate Strings(w557, w556, w555) -> (w553:string)
            n175 = Concatenate Strings(w573, w553) -> (w572:string)
          }
          frame "提取小时数据" {
            n176 = Index Array(array=w596, index (row)=w583) -> (element=w595:string[])  [unwired: 1 in]
            n177 = Index Array(array=w595, index #2=1 ("索引")) -> (element #2=w585:string)  [unwired: 1 in, 1 out]
            n178 = Empty String/Path?(string/path=w585) -> (empty?=w587:bool)
            n179 = case shown="假" w587 {
              tunnel: w585 -> [w601 w603]
              tunnel: w584 -> [w600 _]
              tunnel: [w598 w603] -> w586
              frame False {
                n180 = Fract/Exp String To Number(string=w601) -> (number=w602:dbl)  [unwired: 3 in, 1 out]
                n181 = Multiply(x=w602, y=w600) -> (x*y=w599:dbl)
                n182 = Number To Fractional String(number=w599) -> (F-format string=w598:string)  [unwired: 3 in]
              }
              frame True {
                # "空"
              }
            }
            n183 = call "datacodecomb.vi"("数据标识"="N", "数据类型"="-Avg=", "污染物编码"=w591, "地表水/污染源"=w582, "污染物浓度"=w586) -> ("编码输出"=w590:string)  [unwired: 6 in]
            n184 = case shown="\"2017-212协议\"" w581 {
              tunnel: w591 -> [w606 _]
              tunnel: w590 -> [w604 w609]
              tunnel: [w605 w609] -> w592
              frame "2005-212协议", Default {
                n185 = case shown="\"假\", 默认" w606 {
                  tunnel: [w607 ""] -> w605
                  tunnel: w604 -> [w607 _]
                  frame "假", Default {
                  }
                  frame "累积流量", "流速", "水位" {
                  }
                }
              }
              frame "2017-212协议" {
              }
            }
            n186 = Concatenate Strings(w589, w592) -> (w588:string)
          }
          frame "提取实时数据" {
            n187 = Index Array(array=w619, index (row)=w610) -> (element=w625:string[])  [unwired: 1 in]
            n188 = Index Array(array=w625, index #1=3 ("索引"), index #2=5 ("索引")) -> (element #1=w614:string, element #2=w623:string)
            n189 = Empty String/Path?(string/path=w614) -> (empty?=w616:bool)
            n190 = case shown="假" w616 {
              tunnel: w614 -> [w631 w633]
              tunnel: w613 -> [w630 _]
              tunnel: [w628 w633] -> w615
              frame False {
                n191 = Fract/Exp String To Number(string=w631) -> (number=w632:dbl)  [unwired: 3 in, 1 out]
                n192 = Multiply(x=w632, y=w630) -> (x*y=w629:dbl)
                n193 = Number To Fractional String(number=w629) -> (F-format string=w628:string)  [unwired: 3 in]
              }
              frame True {
                # "空"
              }
            }
            n194 = call "datacodecomb.vi"("数据标识"=w623, "数据类型"="-Rtd=", "污染物编码"=w618, "地表水/污染源"=w612, "污染物浓度"=w615) -> ("编码输出"=w622:string)  [unwired: 6 in]
            n195 = case shown="\"2017-212协议\"" w611 {
              tunnel: w618 -> [w636 _]
              tunnel: w622 -> [w634 w639]
              tunnel: [w635 w639] -> w621
              frame "2005-212协议", Default {
                n196 = case shown="\"累积流量\", \"流速\", \"水位\"" w636 {
                  tunnel: [w637 ""] -> w635
                  tunnel: w634 -> [w637 _]
                  frame "假", Default {
                  }
                  frame "累积流量", "流速", "水位" {
                  }
                }
              }
              frame "2017-212协议" {
              }
            }
            n197 = Concatenate Strings(w620, w621) -> (w617:string)
          }
          frame "操作日志" {
            n198 = Unbundle By Name(w640) -> ("DO"=w646:string)
            n199 = Index Array(array=w655, index (row)=w641) -> (element=w654:string[])  [unwired: 1 in]
            n200 = Equal?(x=w644, y=w646) -> (x = y?=w642:bool)
            n201 = Index Array(array=w654, index #1=0 ("索引"), index #2=2 ("索引")) -> (element #2=w653:string)  [unwired: 1 out]
            n202 = Empty String/Path?(string/path=w653) -> (empty?=w658:bool)
            n203 = Select(t="w00000", s=w642, f=w644) -> (s? t:f=w643:string)
            n204 = Select(t="i21001", s=w642, f="i11001") -> (s? t:f=w647:string)
            n205 = case shown="假" w658 {
              tunnel: [w662 ""] -> w652
              tunnel: w653 -> [w660 _]
              tunnel: w643 -> [w661 _]
              tunnel: w647 -> [w659 _]
              frame False {
                n206 = Format Into String(format string="PolId=%s,%s-Info=//%s//;" ("格式字符串"), w661, w659, w660) -> (resulting string=w662:string)  [unwired: 2 in, 1 out]
              }
              frame True {
              }
            }
            n207 = Concatenate Strings(w651, w652) -> (w650:string)
          }
          frame "仪器参数" {
            n208 = case shown="\"STD\", 默认" w665 {
              tunnel: ["3090仪器参数" ("table") "仪器参数" ("table")] -> w667
              frame "STD", Default {
              }
              frame "GB212" {
              }
            }
            n209 = Index Array(array=w673, index (row)=w666) -> (element=w672:string[])  [unwired: 1 in]
            n210 = call "keyparametercomb.vi"("应用环境"=w665, "table"=w667, "因子编码"=w671, "data"=w672) -> ("字符串"=w670:string)  [unwired: 7 in]
            n211 = Concatenate Strings(w669, w670) -> (w668:string)
          }
          frame "3090仪器参数" {
            n212 = Index Array(array=w681, index (row)=w677) -> (element=w683:string[])  [unwired: 1 in]
            n213 = call "keyparametercomb.vi"("应用环境"=w676, "table"="3090仪器参数", "因子编码"=w679, "data"=w683) -> ("字符串"=w682:string)  [unwired: 7 in]
            n214 = Concatenate Strings(w680, w682) -> (w678:string)
          }
          frame "提取仪器参数" {
            n215 = Index Array(array=w695, index (row)=w692) -> (element=w688:string[])  [unwired: 1 in]
            n216 = Index Array(array=w688, index=0 ("索引")) -> (element=w690:string)
            n217 = Empty String/Path?(string/path=w690) -> (empty?=w691:bool)
            n218 = case shown="假" w691 {
              tunnel: [w701 ""] -> w686
              tunnel: w688 -> [w699 _]
              tunnel: w690 -> [w698 _]
              tunnel: w687 -> [w697 _]
              tunnel: w685 -> [w696 _]
              frame False {
                n219 = Spreadsheet String To Array(delimiter (Tab)="," ("分隔符(Tab)"), format string="" ("格式字符串"), spreadsheet string=w697, array type (2D Dbl)=string[] []) -> (array=w707:string[])
                n220 = for {
                  shift-right: [w718] -> w705
                  shift-left: "" -> [w717]
                  tunnel: w707 -> [w719] mode=indexing
                  tunnel: w699 -> [w715]
                  n221 = case shown="\"i13003\"" w719 {
                    tunnel: [2 ("索引") 3 ("索引") 4 ("索引") 5 ("索引") 6 ("索引") 7 ("索引") 8 ("索引") 9 ("索引") 10 ("索引") 11 ("索引") 12 ("索引") 13 ("索引") 14 ("索引") 15 ("索引") 16 ("索引") 17 ("索引") 18 ("索引") 19 ("索引") 20 ("索引") 21 ("索引") 22 ("索引") 23 ("索引") 24 ("索引") 25 ("索引") 26 ("索引") 27 ("索引") 28 ("索引")] -> w722
                    frame "i13001", Default {
                    }
                    frame "i13002" {
                    }
                    frame "i13003" {
                    }
                    frame "i13004" {
                    }
                    frame "i13005" {
                    }
                    frame "i13006" {
                    }
                    frame "i13007" {
                    }
                    frame "i13008" {
                    }
                    frame "i13009" {
                    }
                    frame "i13010" {
                    }
                    frame "i13011" {
                    }
                    frame "i13012" {
                    }
                    frame "i13013" {
                    }
                    frame "i13014" {
                    }
                    frame "i13015" {
                    }
                    frame "i13016" {
                    }
                    frame "i13017" {
                    }
                    frame "i13101" {
                    }
                    frame "i13102" {
                    }
                    frame "i13103" {
                    }
                    frame "i13104" {
                    }
                    frame "i13105" {
                    }
                    frame "i13106" {
                    }
                    frame "i13107" {
                    }
                    frame "i13108" {
                    }
                    frame "i13109" {
                    }
                    frame "i13110" {
                    }
                  }
                  n222 = Concatenate Strings(w719, "-Info=%s," ("格式字符串")) -> (w713:string)
                  n223 = Index Array(array=w715, index #1=0 ("索引"), index #2=w722) -> (element #2=w720:string)  [unwired: 1 out]
                  n224 = case shown="\"i13006\", \"i13013\"" w719 {
                    tunnel: w720 -> [w724 w728]
                    tunnel: [w723 w727] -> w712
                    frame "假", Default {
                      n225 = Fract/Exp String To Number(string=w724) -> (number=w725:dbl)  [unwired: 3 in, 1 out]
                      n226 = Number To Fractional String(number=w725, precision (6)=i16 6 ("精度(6)")) -> (F-format string=w723:string)  [unwired: 2 in]
                    }
                    frame "i13006", "i13013" {
                      n227 = call "formatstringtime.vi"("字符串"=w728) -> ("result string"=w727:string)  [unwired: 10 in]
                    }
                  }
                  n228 = Format Into String(format string=w713, w712) -> (resulting string=w716:string)  [unwired: 2 in, 1 out]
                  n229 = Concatenate Strings(w717, w716) -> (w718:string)
                }
                n230 = call "formatstringtime.vi"("字符串"=w698) -> ("result string"=w700:string)  [unwired: 10 in]
                n231 = String Length(string=w705) -> (length=w704:i32)
                n232 = Decrement(x=w704) -> (x-1=w703:i32)
                n233 = String Subset(string=w705, length (rest)=w703) -> (substring=w702:string)  [unwired: 1 in]
                n234 = Format Into String(format string="DataTime=%s;PolId=%s,%s" ("格式字符串"), w700, w696, w702) -> (resulting string=w701:string)  [unwired: 2 in, 1 out]
              }
              frame True {
              }
            }
            n235 = Concatenate Strings(w694, w686) -> (w693:string)
          }
          frame "报警信息" {
            n236 = case shown="\"CODCr\"" w779 {
              tunnel: [u16 0 ("register") w804 w810 w816 w822 w828] -> w777
              tunnel: [u16 0 ("register") w802 w808 w814 w820 w826] -> w761
              tunnel: w758 -> [_ w801 w807 w813 w819 w825]
              tunnel: w757 -> [_ w800 w806 w812 w818 w824]
              frame "假", Default {
              }
              frame "CODMn" {
                n237 = Index Array(array=w801, index=1 ("索引")) -> (element=w804:u16)
                n238 = Index Array(array=w800, index=1 ("索引")) -> (element=w802:u16)
              }
              frame "氨氮" {
                n239 = Index Array(array=w807, index=2 ("索引")) -> (element=w810:u16)
                n240 = Index Array(array=w806, index=2 ("索引")) -> (element=w808:u16)
              }
              frame "总磷" {
                n241 = Index Array(array=w813, index=3 ("索引")) -> (element=w816:u16)
                n242 = Index Array(array=w812, index=3 ("索引")) -> (element=w814:u16)
              }
              frame "总氮" {
                n243 = Index Array(array=w819, index=4 ("索引")) -> (element=w822:u16)
                n244 = Index Array(array=w818, index=4 ("索引")) -> (element=w820:u16)
              }
              frame "CODCr" {
                n245 = Index Array(array=w825, index=5 ("索引")) -> (element=w828:u16)
                n246 = Index Array(array=w824, index=5 ("索引")) -> (element=w826:u16)
              }
            }
            n247 = Unbundle By Name(w759) -> ("藻密度"=w785:string)
            n248 = Empty String/Path?(string/path=w764) -> (empty?=w763:bool)
            n249 = Index Array(array=w781, index (row)=w760) -> (element=w780:string[])  [unwired: 1 in]
            n250 = Equal?(x=w783, y=w785) -> (x = y?=w774:bool)
            n251 = Select(t="w00000", s=w774, f=w783) -> (s? t:f=w782:string)
            n252 = Index Array(array=w780, index #1=0 ("索引"), index #2=2 ("索引")) -> (element #1=w771:string, element #2=w791:string)
            n253 = Empty String/Path?(string/path=w791) -> (empty?=w790:bool)
            n254 = Select(t="i22001", s=w774, f="i12001") -> (s? t:f=w773:string)
            n255 = Select(t="i22003", s=w774, f="i12031") -> (s? t:f=w772:string)
            n256 = Number To Decimal String(number=w777) -> (decimal integer string=w778:string)  [unwired: 1 in]
            n257 = Number To Decimal String(number=w761) -> (decimal integer string=w762:string)  [unwired: 1 in]
            n258 = case shown="假" w790 {
              tunnel: [w838 ""] -> w768
              tunnel: w791 -> [w835 _]
              tunnel: w782 -> [w833 _]
              tunnel: w778 -> [w831 _]
              tunnel: w773 -> [w832 _]
              tunnel: w772 -> [w836 _]
              tunnel: w762 -> [w830 _]
              frame False {
                n259 = call "alarmtexttoi12031.vi"("字符串"=w835) -> ("十进制整型字符串"=w834:string)  [unwired: 10 in]
                n260 = Format Into String(format string="PolId=%s,%s-Info=%s,i12002-Info=0,i12003-Info=%s,%s-Info=%s;" ("格式字符串"), w833, w832, w831, w830, w836, w834) -> (resulting string=w838:string)  [unwired: 2 in, 1 out]
              }
              frame True {
              }
            }
            n261 = Empty String/Path?(string/path=w768) -> (empty?=w767:bool)
            n262 = Concatenate Strings(w764, w768) -> (w770:string)
            n263 = Not(x=w767) -> (.not. x?=w766:bool)
            n264 = And(x=w763, y=w766) -> (x .and. y?=w765:bool)
            n265 = case shown="真" w765 {
              tunnel: w771 -> [_ w795]
              tunnel: w770 -> [w792 w794]
              tunnel: [w792 w793] -> w769
              frame False {
              }
              frame True {
                n266 = call "formatstringtime.vi"("字符串"=w795) -> ("result string"=w797:string)  [unwired: 10 in]
                n267 = Format Into String(format string="DataTime=%s;%s", w797, w794) -> (resulting string=w793:string)  [unwired: 2 in, 1 out]
              }
            }
          }
        }
      }
    }
    frame Error {
    }
  }
  "error out" <- w5
  "object out" <- w3
  "字符串" <- w1
